vi "Format MonitorInstancesResult_LVXML_InstancesSet.vi"(8 "error in (no error)":errorcluster, 11 "Siblings":T3(array[cluster])) -> (0 "error out":errorcluster, 3 "Array":T1(array[cluster]))   [LabVIEW 2014, in "AWS_EC2.lvlib" / "AWS_EC2.lvclass"]
uses:
  AWS_EC2.lvclass
  lv-xml-parser/r0/trunk/VI Source/EventType.ctl
  lv-xml-parser/r0/trunk/VI Source/LV XML Parser.lvlib
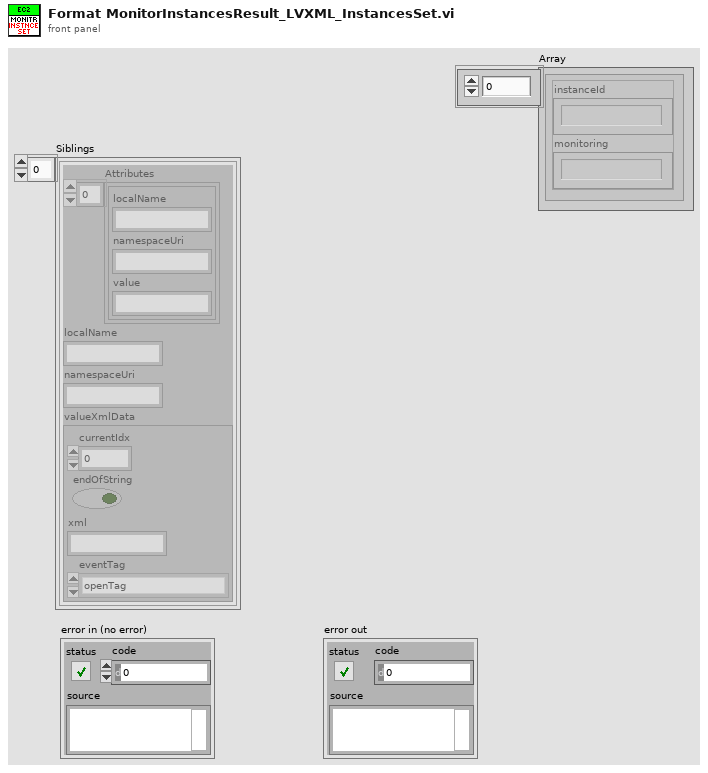
[diagram p1: front panel]
types:
  T1 = cluster{"instanceId":string, "monitoring":string}[]
  T2 = typedef "LV XML Parser.lvlib/EventType.ctl" = enum16{"openTag", "endOpenTag", "closeTag", "comment", "endComment", "endOfFile", "attribute", "startXml"}
  T3 = cluster{"Attributes":cluster{"localName":string, "namespaceUri":string, "value":string}[], "localName":string, "namespaceUri":string, "valueXmlData":cluster{"currentIdx":i32, "endOfString":bool, "xml":string, "eventTag":T2}}[]
  T4 = cluster{"Attributes":cluster{"localName":string, "namespaceUri":string, "value":string}[], "localName":string, "namespaceUri":string, "valueXmlData":cluster{"currentIdx":i32, "endOfString":bool, "xml":string, "eventTag":T2}}
  T5 = cluster{"currentIdx":i32, "endOfString":bool, "xml":string, "eventTag":T2}
  T6 = cluster{"namespaceUri":string, "localName":string}
  T7 = cluster{"instanceId":string, "monitoring":string}
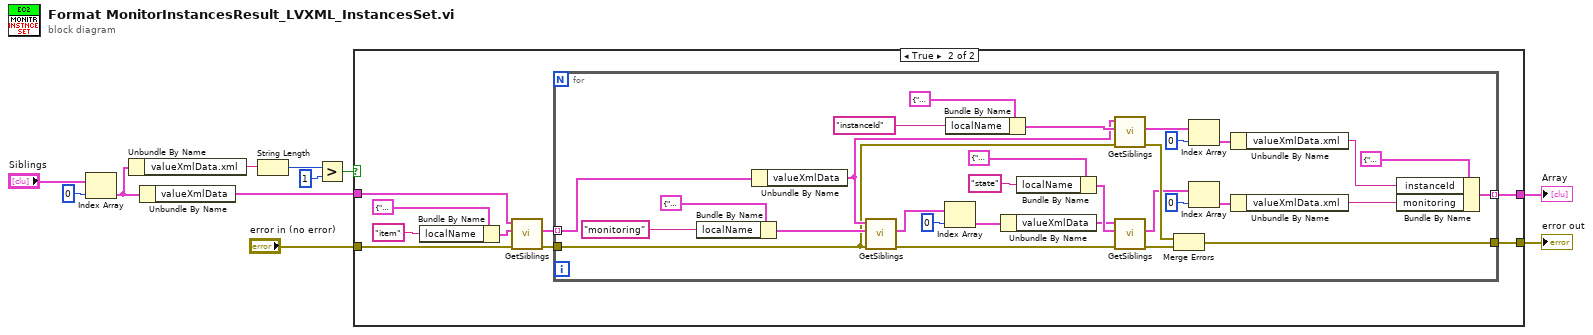
[diagram p0: block diagram]
diagram:
  n1 = Index Array(array="Siblings", index=0) -> (element=w2:T4)
  n2 = Unbundle By Name(w2) -> ("valueXmlData.xml"=w3:string)
  n3 = Unbundle By Name(w2) -> ("valueXmlData"=w4:T5)
  n4 = String Length(string=w3) -> (length=w7:i32)
  n5 = Greater?(x=w7, y=1) -> (0:w5:bool)
  n6 = case shown="True" w5 {
    tunnel: [w12 w20] -> w11
    tunnel: [_ w19] -> w1
    tunnel: "error in (no error)" -> [w12 w14]
    tunnel: w4 -> [_ w13]
    frame False {
    }
    frame True {
      n7 = Bundle By Name(cluster=T6 {"namespaceUri"="", "localName"=""} ("limitToTag"), "localName"="item" ("Tag name")) -> (w16:T6)
      n8 = call "GetSiblings.vi"("error in (no error)"=w14, "limitToTag"=w16, "xmlData"=w13) -> ("error out"=w21:errorcluster, "Siblings"=w17:T3)  [unwired: 7 in]
      n9 = for {
        tunnel: w17 -> [w45] mode=indexing
        tunnel: [w43] -> w19 mode=indexing
        tunnel: [w44] -> w20
        tunnel: w21 -> [w33]
        n10 = Bundle By Name(cluster=T6 {"namespaceUri"="", "localName"=""} ("limitToTag"), "localName"="monitoring" ("Tag name")) -> (w37:T6)
        n11 = Unbundle By Name(w45) -> ("valueXmlData"=w34:T5)
        n12 = call "GetSiblings.vi"("error in (no error)"=w33, "limitToTag"=w37, "xmlData"=w34) -> ("error out"=w29:errorcluster, "Siblings"=w39:T3)  [unwired: 7 in]
        n13 = Index Array(array=w39, index=0) -> (element=w40:T4)
        n14 = Bundle By Name(cluster=T6 {"namespaceUri"="", "localName"=""} ("limitToTag"), "localName"="instanceId" ("Tag name")) -> (w49:T6)
        n15 = Unbundle By Name(w40) -> ("valueXmlData"=w26:T5)
        n16 = Bundle By Name(cluster=T6 {"namespaceUri"="", "localName"=""} ("limitToTag"), "localName"="state" ("Tag name")) -> (w27:T6)
        n17 = call "GetSiblings.vi"("error in (no error)"=w33, "limitToTag"=w49, "xmlData"=w34) -> ("error out"=w32:errorcluster, "Siblings"=w47:T3)  [unwired: 7 in]
        n18 = call "GetSiblings.vi"("error in (no error)"=w29, "limitToTag"=w27, "xmlData"=w26) -> ("error out"=w28:errorcluster, "Siblings"=w23:T3)  [unwired: 7 in]
        n19 = Merge Errors(w32, w28) -> (w44:errorcluster)
        n20 = Index Array(array=w47, index=0) -> (element=w46:T4)
        n21 = Index Array(array=w23, index=0) -> (element=w24:T4)
        n22 = Unbundle By Name(w46) -> ("valueXmlData.xml"=w41:string)
        n23 = Unbundle By Name(w24) -> ("valueXmlData.xml"=w22:string)
        n24 = Bundle By Name(cluster=T7 {"instanceId"="", "monitoring"=""} ("MonitorInstanceReponseSetItemType"), "instanceId"=w41, "monitoring"=w22) -> (w43:T7)
      }
    }
  }
  "error out" <- w11
  "Array" <- w1
